vi "参数配置表.vi"() -> ()   [LabVIEW 2016, in "数据传输系统-03.lvlib"]
uses:
  <vilib>/Utility/miscctls.llb/LVPointTypeDef.ctl
  <vilib>/Utility/config.llb/NI_LVConfig.lvlib
  <vilib>/ptbypt/NI_PtbyPt.lvlib
panel:
  in  "数据库类型":enum16{"Access", "SQLite"}(ring)
  in  "应用环境":enum16{"STD", "GB212"}(ring)
  in  "屏蔽维护数据":bool
  in  "数据发送延时时间/s":i32
  in  "判断数据反馈":enum16{"非严格判断", "严格判断", "不判断"}(ring)
  in  "仪器参数发送":bool
  in  "地表水/污染源":bool
  in  "间隔时间/分钟":i32
  in  "数据发送通道":enum16{"TCP", "VISA"}(ring)
  in  "数据发送协议":enum16{"2005-212协议", "2017-212协议"}(ring)=enum."2017-212协议"
  in  "数据触发上传方式":enum16{"出数即刻发送", "间隔时间发送", "整点发送"}(ring)
  in  "数据组合发送":bool
  in  "日志、参数发送":bool
  in  "2011发送":bool
  in  "返回":bool
  out "配置表格":string[][](table)
  in  "参数数值":T1={"CODMn"=TRUE, "CODCr"=TRUE, "DO"=TRUE, "铜"=TRUE, "PH"=TRUE, "氨氮"=TRUE, "比电导率"=TRUE, "水温"=TRUE, "COD"=TRUE, "浊度"=TRUE, "总氮"=TRUE, "总磷"=TRUE, "叶绿素a"=TRUE, "藻密度"=TRUE, "水位"=TRUE, "流速"=TRUE, "瞬时流量"=TRUE, "累积流量"=TRUE, "亚硝氮"=TRUE, "硫化物"=TRUE, "ORP"=TRUE, "铅"=TRUE, "镉"=TRUE, "锌"=TRUE, "镍"=TRUE, "锰"=TRUE, "汞"=TRUE, "气温"=TRUE, "气压"=TRUE, "风速"=TRUE, "风向"=TRUE, "盐度"=TRUE, "磷酸盐"=TRUE, "硝氮"=TRUE}
  # "因子编码，单位配置，上传功能码，小时、质控数据上传触发方式"
  # "参数配置"
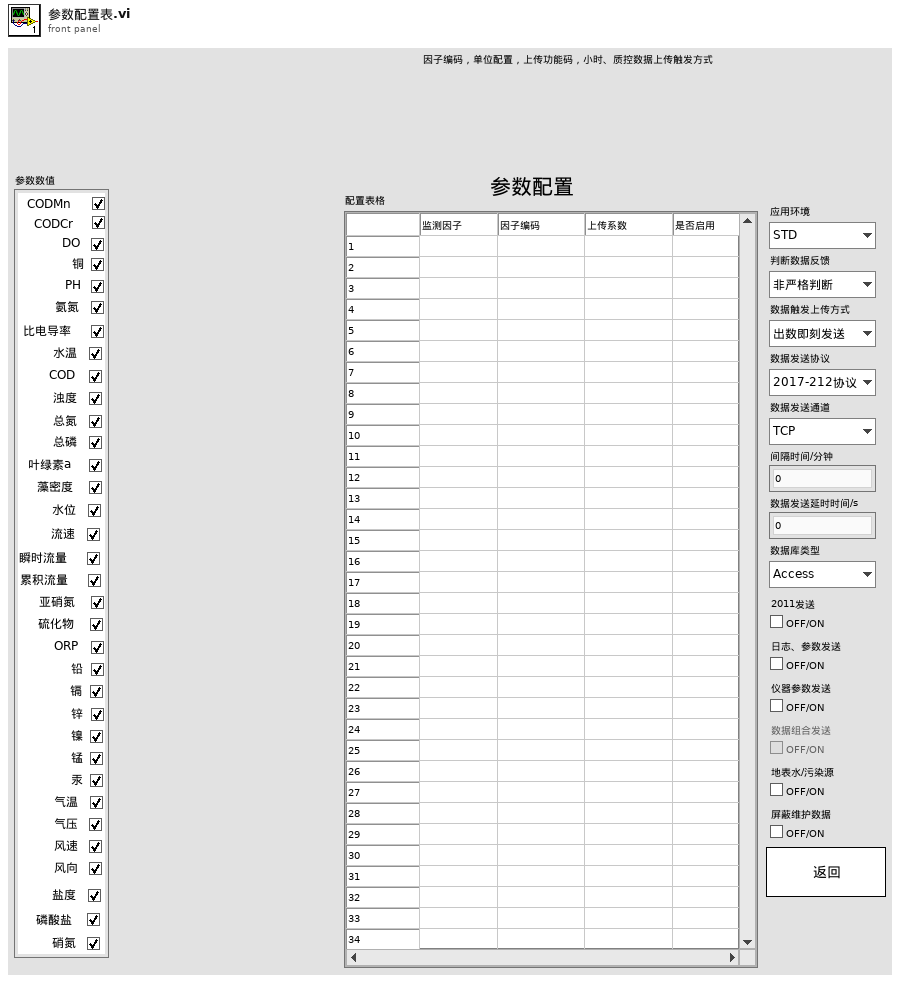
[diagram p1: front panel]
types:
  T1 = cluster{"CODMn":bool, "CODCr":bool, "DO":bool, "铜":bool, "PH":bool, "氨氮":bool, "比电导率":bool, "水温":bool, "COD":bool, "浊度":bool, "总氮":bool, "总磷":bool, "叶绿素a":bool, "藻密度":bool, "水位":bool, "流速":bool, "瞬时流量":bool, "累积流量":bool, "亚硝氮":bool, "硫化物":bool, "ORP":bool, "铅":bool, "镉":bool, "锌":bool, "镍":bool, "锰":bool, "汞":bool, "气温":bool, "气压":bool, "风速":bool, "风向":bool, "盐度":bool, "磷酸盐":bool, "硝氮":bool}
  T2 = typedef "LVPointTypeDef.ctl" = cluster{"Horizontal":i16, "Vertical":i16}
  T3 = typedef "NI_LVConfig.lvlib/Config Data RefNum.ctl" = refnum<k1>
  T4 = cluster{"[0]":string, "[1]":string, "[2]":string, "[3]":string, "[4]":string, "[5]":string, "[6]":string, "[7]":string, "[8]":string, "[9]":string, "[10]":string, "[11]":string, "[12]":string, "[13]":string, "[14]":string, "[15]":string, "[16]":string, "[17]":string, "[18]":string, "[19]":string, "[20]":string, "[21]":string, "[22]":string, "[23]":string, "[24]":string, "[25]":string, "[26]":string, "[27]":string, "[28]":string, "[29]":string, "[30]":string, "[31]":string, "[32]":string, "[33]":string}
  T5 = enum8{"Enabled", "Disabled", "Disabled and Grayed Out"}
  T6 = typedef "LVRowAndColumnTypeDef.ctl" = cluster{"Row":i32, "Column":i32}
  T7 = cluster{"[0]":string, "[1]":string, "[2]":string, "[3]":string, "[4]":string, "[5]":string}
  T8 = cluster{"[0]":string, "[1]":string, "[2]":string, "[3]":string, "[4]":string, "[5]":string, "[6]":string, "[7]":string, "[8]":string, "[9]":string, "[10]":string, "[11]":string}
  T9 = cluster{"[0]":string, "[1]":string, "[2]":string, "[3]":string, "[4]":string, "[5]":string, "[6]":string, "[7]":string, "[8]":string, "[9]":string, "[10]":string, "[11]":string, "[12]":string}
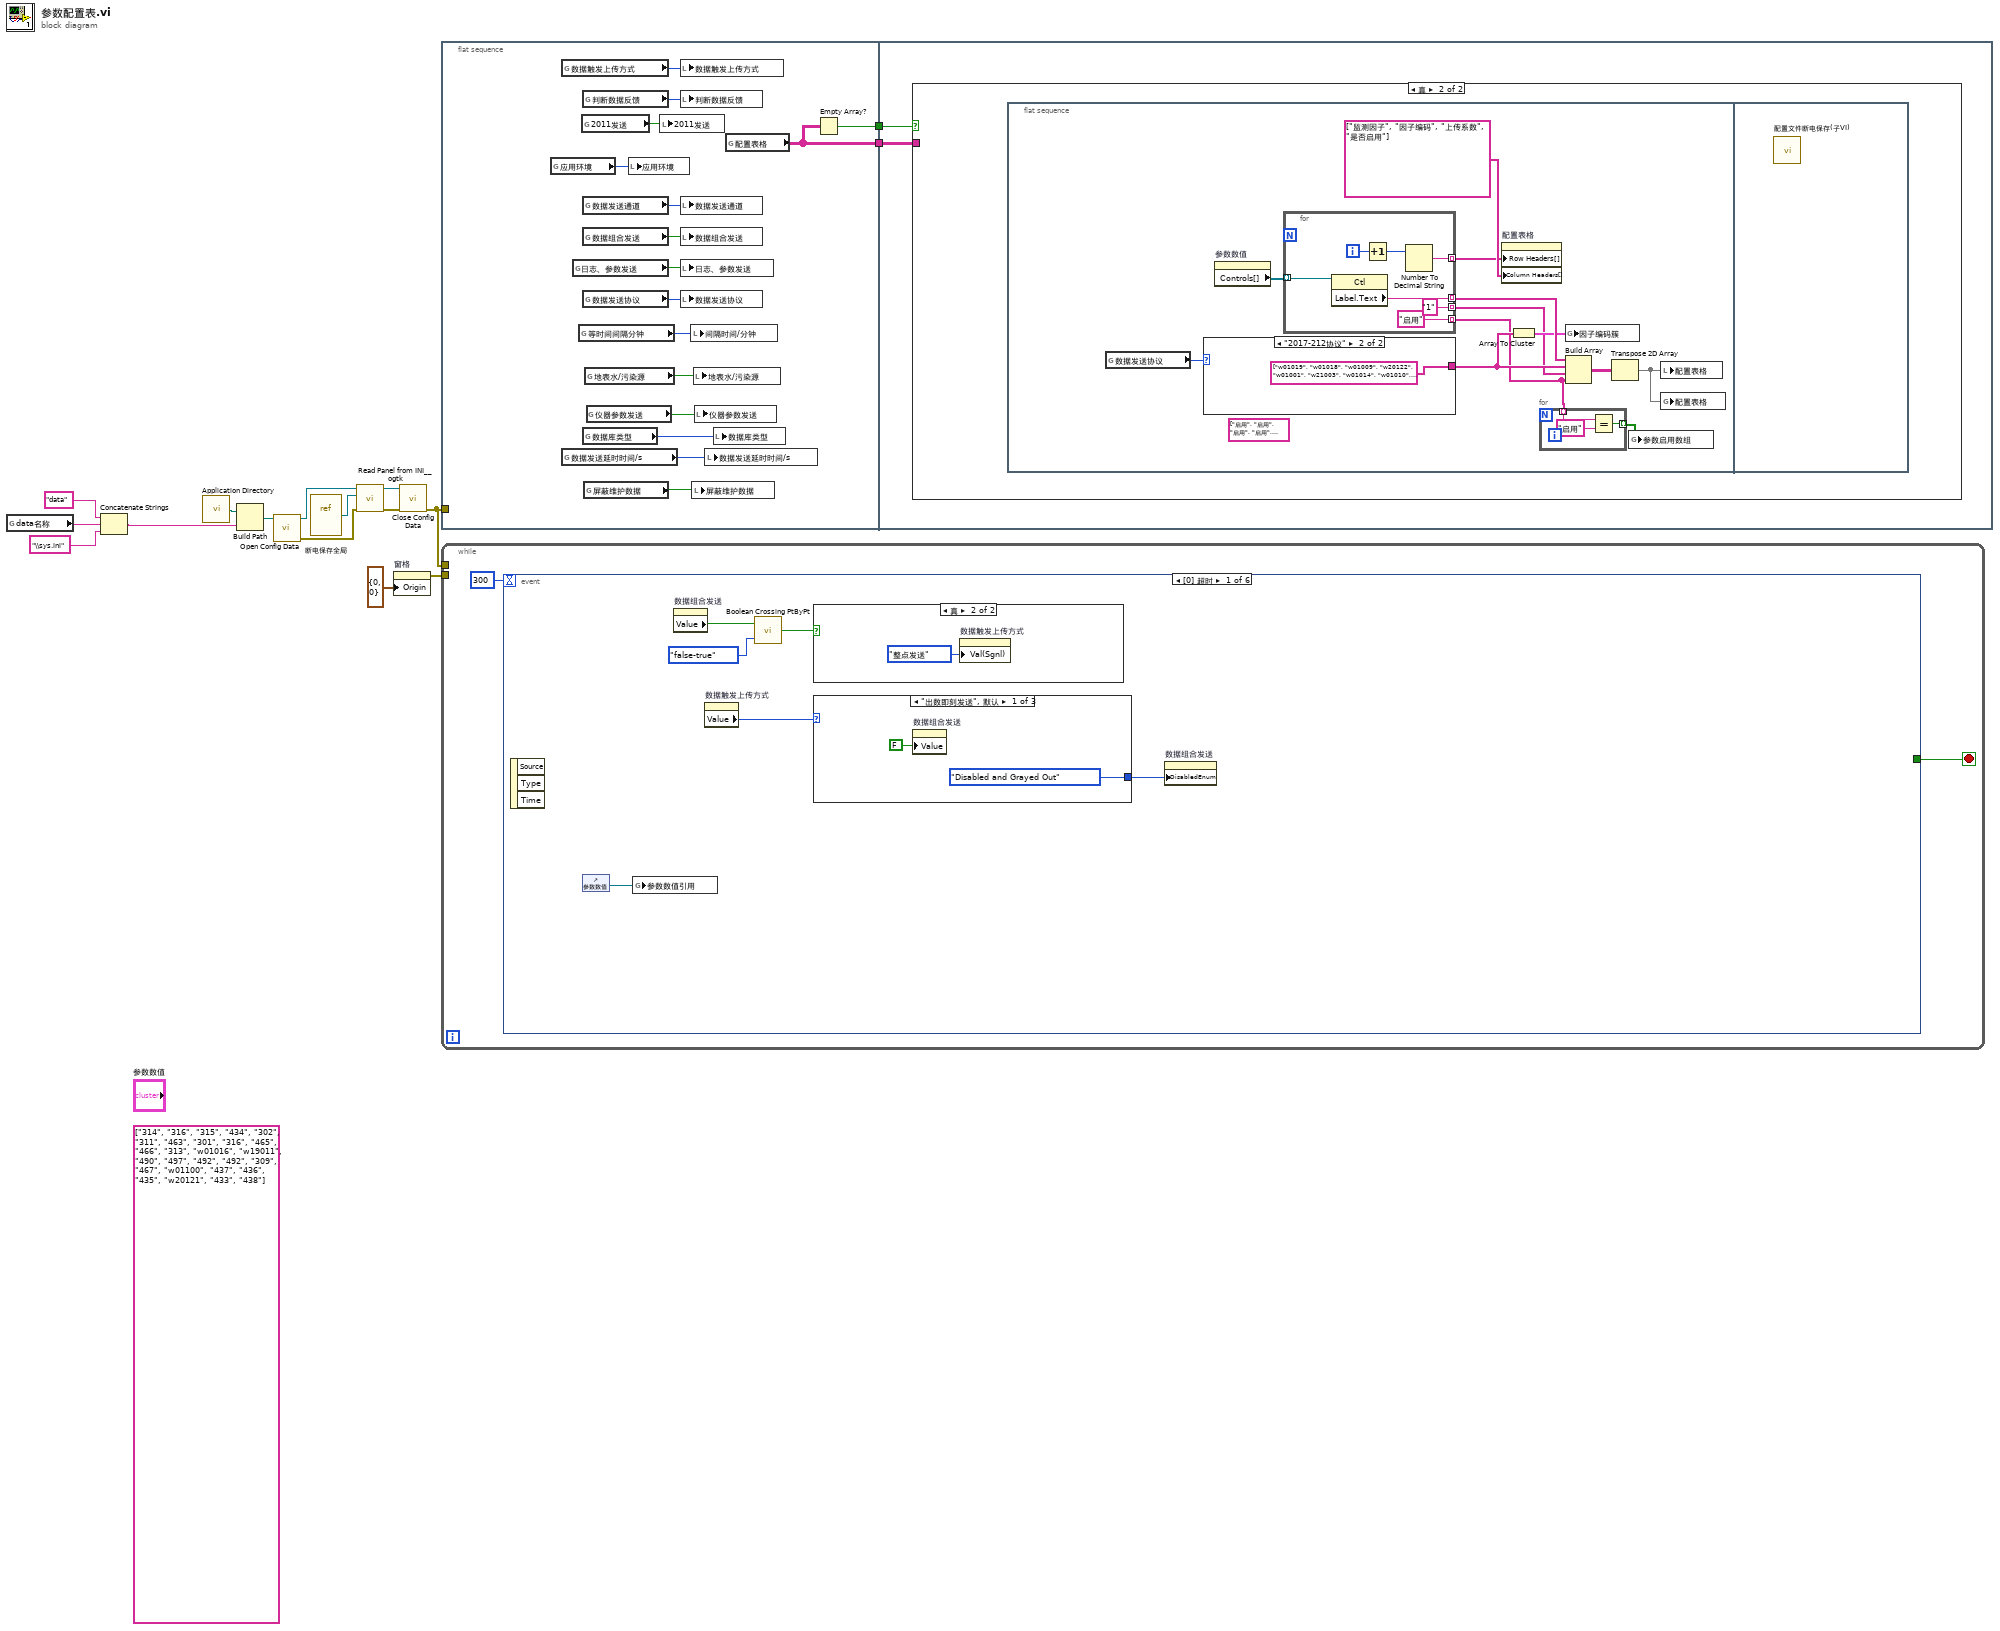
[diagram p0: block diagram]
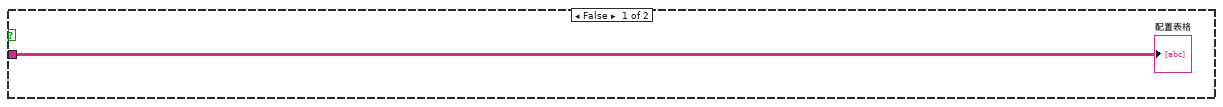
[diagram p2: hidden frame]
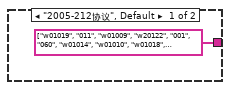
[diagram p3: hidden frame]
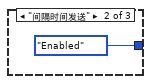
[diagram p5: hidden frame]
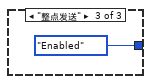
[diagram p6: hidden frame]
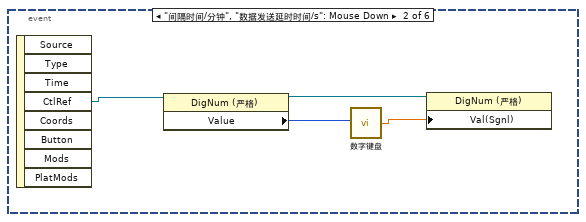
[diagram p7: hidden frame]
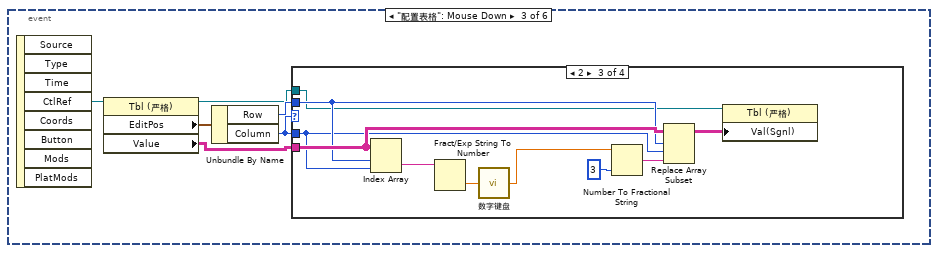
[diagram p8: hidden frame]
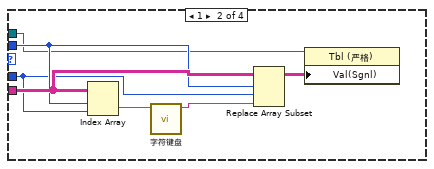
[diagram p10: hidden frame]
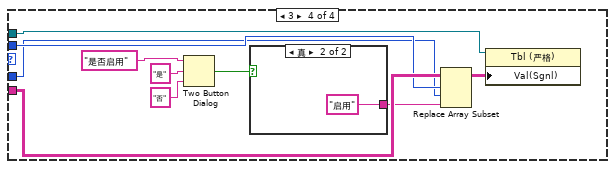
[diagram p11: hidden frame]
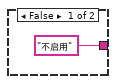
[diagram p12: hidden frame]
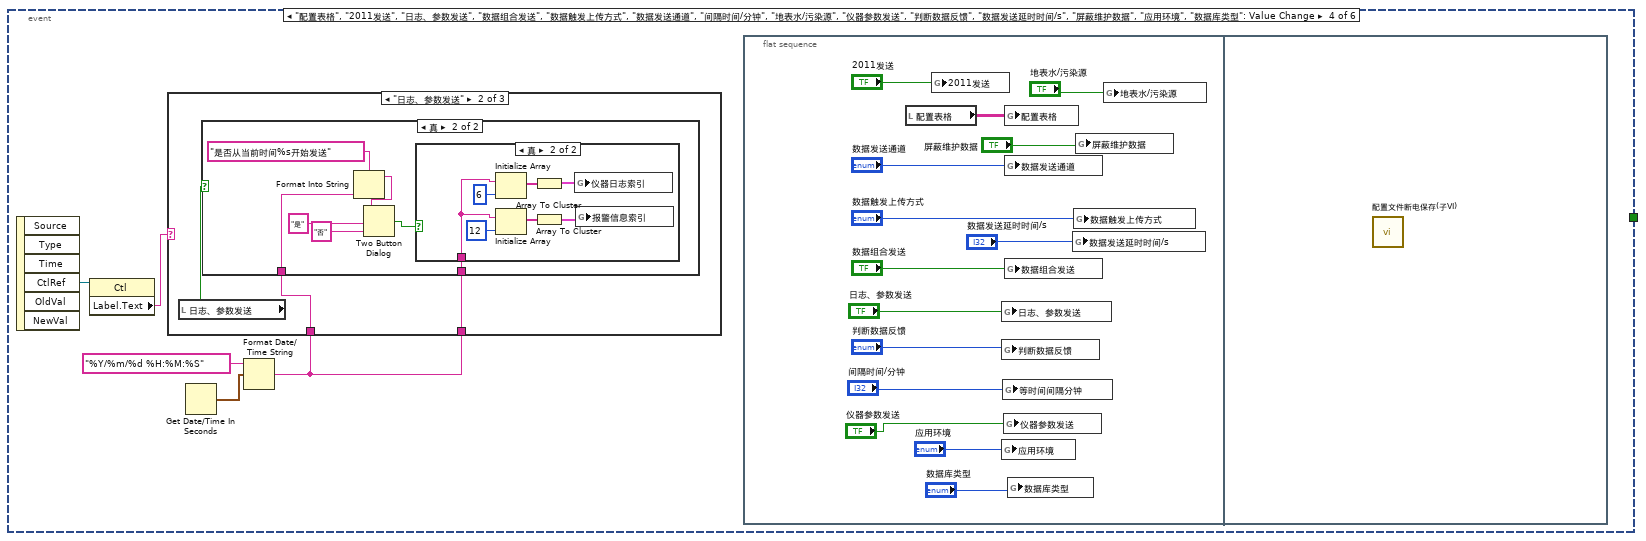
[diagram p13: hidden frame]
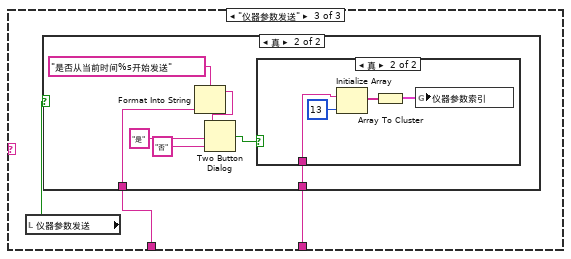
[diagram p17: hidden frame]
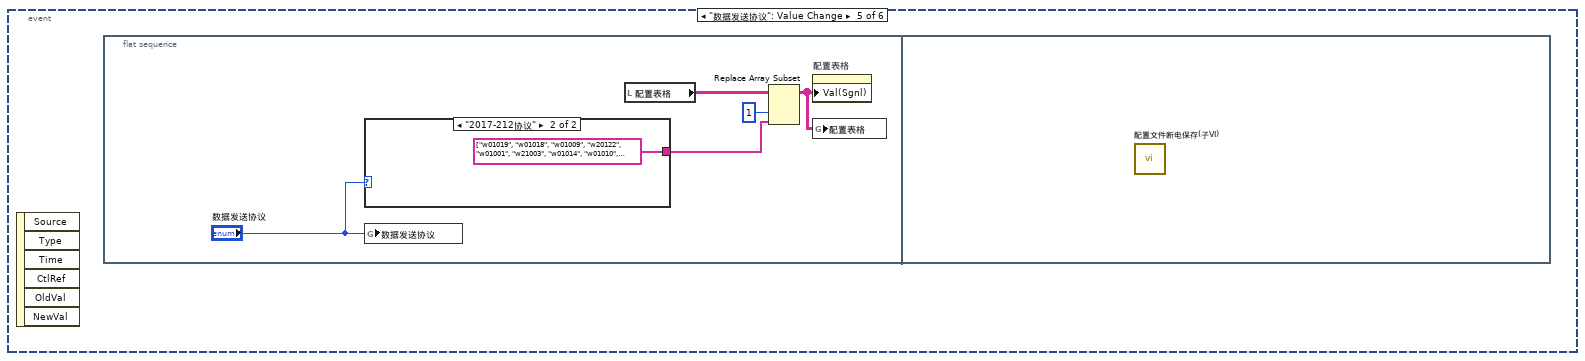
[diagram p20: hidden frame]
diagram:
  (unwired) string[] ["314", "316", "315", "434", "302", "311", "463", "301", "316", "465", "466", "313", "w01016", "w19011", "490", "497", "492", "492", "309", "467", "w01100", "437", "436", "435", "w20121", "433", "438"]
  n1 = global read "断电保存全局.vi" "data名称"() -> (w3:string)
  n2 = Concatenate Strings("data" ("名称或相对路径"), w3, "\\sys.ini" ("名称或相对路径")) -> (w1:string)
  n3 = call <vilib>:"Application Directory.vi"() -> ("Application Directory"=w12:path)
  n4 = Build Path(base path=w12, name or relative path=w1) -> (appended path=w11:path)
  n5 = call <vilib>:"Open Config Data.vi"("configuration file path"=w11) -> ("error out"=w16:errorcluster, "refnum"=w15:T3)  [unwired: 8 in, 1 out]
  n6 = vi-ref "断电保存全局.vi"() -> (w14:refnum<vi>)
  n7 = call <userlib>:"Read Panel from INI__ogtk.vi"("error in (no error)"=w16, "VI ref"=w14, "refnum"=w15) -> ("error out"=w10:errorcluster, "refnum out"=w13:T3)  [unwired: 7 in]
  n8 = property on="窗格" class="Pane"("Origin"=T2 {"Horizontal"=0, "Vertical"=0} ("原点")) -> (error out=w8:errorcluster)  [unwired: 2 in, 1 out]
  n9 = call <vilib>:"Close Config Data.vi"("error in (no error)"=w10, "refnum"=w13) -> ("error out"=w9:errorcluster)  [unwired: 8 in, 1 out]
  n10 = flat-sequence {
    tunnel: w9 -> [_]
    tunnel: [w25] -> w6
    tunnel: [w24] -> w5
    tunnel: w6 -> [w34]
    tunnel: w5 -> [w33]
    frame #0 {
      n11 = global read "断电保存全局.vi" "应用环境"() -> (w18:enum16{"STD", "GB212"})
      n12 = global read "断电保存全局.vi" "数据触发上传方式"() -> (w28:enum16{"出数即刻发送", "间隔时间发送", "整点发送"})
      n13 = global read "断电保存全局.vi" "数据发送延时时间/s"() -> (w20:i32)
      n14 = global read "断电保存全局.vi" "日志、参数发送"() -> (w30:bool)
      n15 = global read "断电保存全局.vi" "等时间间隔分钟"() -> (w23:i32)
      n16 = global read "断电保存全局.vi" "2011发送"() -> (w32:bool)
      n17 = global read "断电保存全局.vi" "判断数据反馈"() -> (w31:enum16{"非严格判断", "严格判断", "不判断"})
      n18 = global read "断电保存全局.vi" "数据发送通道"() -> (w27:enum16{"TCP", "VISA"})
      n19 = global read "断电保存全局.vi" "数据组合发送"() -> (w29:bool)
      n20 = global read "断电保存全局.vi" "数据发送协议"() -> (w26:enum16{"2005-212协议", "2017-212协议"})
      n21 = global read "断电保存全局.vi" "数据库类型"() -> (w17:enum16{"Access", "SQLite"})
      n22 = global read "断电保存全局.vi" "屏蔽维护数据"() -> (w19:bool)
      n23 = global read "断电保存全局.vi" "地表水/污染源"() -> (w22:bool)
      n24 = global read "断电保存全局.vi" "仪器参数发送"() -> (w21:bool)
      n25 = local write "应用环境"(w18) -> ()
      n26 = local write "2011发送"(w32) -> ()
      n27 = local write "数据触发上传方式"(w28) -> ()
      n28 = local write "判断数据反馈"(w31) -> ()
      n29 = local write "数据发送通道"(w27) -> ()
      n30 = local write "数据组合发送"(w29) -> ()
      n31 = local write "日志、参数发送"(w30) -> ()
      n32 = local write "数据发送协议"(w26) -> ()
      n33 = local write "间隔时间/分钟"(w23) -> ()
      n34 = local write "屏蔽维护数据"(w19) -> ()
      n35 = local write "地表水/污染源"(w22) -> ()
      n36 = local write "仪器参数发送"(w21) -> ()
      n37 = local write "数据发送延时时间/s"(w20) -> ()
      n38 = local write "数据库类型"(w17) -> ()
      n39 = global read "断电保存全局.vi" "配置表格"() -> (w24:string[][])
      n40 = Empty Array?(array=w24) -> (empty?=w25:bool)
    }
    frame #1 {
      n41 = case shown="真" w34 {
        tunnel: w33 -> [w35 _]
        frame False {
          "配置表格" <- w35
        }
        frame True {
          n42 = flat-sequence {
            frame #0 {
              (unwired) string[] ["启用", "启用", "启用", "启用", "启用", "启用", "启用", "启用", "启用", "启用", "启用", "启用", "启用", "启用", "启用", "启用", "启用", "启用", "启用", "启用", "启用", "启用", "启用", "启用", "启用", "启用", "启用"]
              n43 = global read "断电保存全局.vi" "数据发送协议"() -> (w41:enum16{"2005-212协议", "2017-212协议"})
              n44 = case shown="\"2017-212协议\"" w41 {
                tunnel: [string[] ["w01019", "011", "w01009", "w20122", "001", "060", "w01014", "w01010", "w01018", "w01003", "065", "101", "w01016", "w19011", "e01201", "e01202", "B01", "e01204", "w21006", "w21019", "w01100", "w20120", "w20115", "w20123", "w20121", "w20124", "w20111"] string[] ["w01019", "w01018", "w01009", "w20122", "w01001", "w21003", "w01014", "w01010", "w01018", "w01003", "w21001", "w21011", "w01016", "w19011", "e01201", "e01202", "e01203", "e01204", "w21006", "w21019", "w01100", "w20120", "w20115", "w20123", "w20121", "w20124", "w20111", "a01001", "a01006", "a01007", "a01008", "w01002", "w21015", "w21007"]] -> w39
                frame "2005-212协议", Default {
                }
                frame "2017-212协议" {
                }
              }
              n45 = property on="参数数值" class="Clust (严格)"() -> ("Controls[]"=w43:refnum<vi>[])  [unwired: 2 in, 2 out]
              n46 = for {
                tunnel: w43 -> [w59] mode=indexing
                tunnel: [w58] -> w45 mode=indexing
                tunnel: [w56] -> w44 mode=indexing
                tunnel: ["1"] -> w38 mode=indexing
                tunnel: ["启用"] -> w36 mode=indexing
                i -> [w57]
                n47 = property class="Ctl"(reference=w59) -> ("Label.Text"=w58:string)  [unwired: 1 in, 2 out]
                n48 = Increment(x=w57) -> (x+1=w55:i32)
                n49 = Number To Decimal String(number=w55) -> (decimal integer string=w56:string)  [unwired: 1 in]
              }
              n50 = property on="配置表格" class="Tbl (严格)"("Row Headers[]"=w44, "Column Headers[]"=string[] ["监测因子", "因子编码", "上传系数", "是否启用"]) -> ()  [unwired: 2 in, 2 out]
              n51 = Array To Cluster(array=w39) -> (cluster=w40:T4)
              n52 = for {
                tunnel: w36 -> [w50] mode=indexing
                tunnel: [w48] -> w37 mode=indexing
                n53 = Equal?(x=w50, y="启用") -> (x = y?=w48:bool)
              }
              n54 = global write "断电保存全局.vi" "因子编码簇"(w40) -> ()
              n55 = Build Array(w45, w39, w38, w36) -> (w47:string[][])
              n56 = Transpose 2D Array(2D array=w47) -> (transposed array=w42:string[][])
              n57 = global write "断电保存全局.vi" "参数启用数组"(w37) -> ()
              n58 = local write "配置表格"(w42) -> ()
              n59 = global write "断电保存全局.vi" "配置表格"(w42) -> ()
            }
            frame #1 {
              n60 = call "配置文件断电保存(子VI).vi"() -> ()  [unwired: 12 in]
            }
          }
        }
      }
    }
  }
  n61 = while {
    tunnel: w9 -> [_]
    tunnel: w8 -> [_]
    stop <- w60 stop-if-true
    n62 = event shown="[0] 超时" {
      selector: _ -> [_ _ _ _ _ _]
      dyn-events: _ -> [_ _ _ _ _ _]
      timeout: 300 -> [_ _ _ _ _ _]
      tunnel: [_ _ _ _ _ TRUE] -> w60
      event Timeout {
        n63 = event-data() -> ()  [unwired: 1 in, 3 out]
        n64 = control-ref of="参数数值"() -> (w62:refnum<vi>)
        n65 = global write "断电保存全局.vi" "参数数值引用"(w62) -> ()
        n66 = property on="数据组合发送" class="Bool (严格)"() -> ("Value"=w65:bool)  [unwired: 2 in, 2 out]
        n67 = property on="数据触发上传方式" class="Enum (严格)"() -> ("Value"=w67:enum16{"出数即刻发送", "间隔时间发送", "整点发送"})  [unwired: 2 in, 2 out]
        n68 = call <vilib>:"Boolean Crossing PtByPt.vi"("direction"=enum16{"either", "false-true", "true-false"}."false-true", "input"=w65) -> ("crossing"=w63:bool)  [unwired: 1 in]
        n69 = case shown="真" w63 {
          frame False {
          }
          frame True {
            n70 = property on="数据触发上传方式" class="Enum (严格)"("Val(Sgnl)"=enum16{"出数即刻发送", "间隔时间发送", "整点发送"}."整点发送" ("值(信号)")) -> ()  [unwired: 2 in, 2 out]
          }
        }
        n71 = case shown="\"出数即刻发送\", 默认" w67 {
          tunnel: [T5."Disabled and Grayed Out" ("禁用") T5."Enabled" ("禁用") T5."Enabled" ("禁用")] -> w66
          frame "出数即刻发送", Default {
            n72 = property on="数据组合发送" class="Bool (严格)"("Value"=FALSE ("值(信号)")) -> ()  [unwired: 2 in, 2 out]
          }
          frame "间隔时间发送" {
          }
          frame "整点发送" {
          }
        }
        n73 = property on="数据组合发送" class="Bool (严格)"("DisabledEnum"=w66) -> ()  [unwired: 2 in, 2 out]
      }
      event "间隔时间/分钟", "数据发送延时时间/s": Mouse Down {
        n74 = event-data() -> ("CtlRef"=w76:refnum<vi>)  [unwired: 1 in, 7 out]
        n75 = property class="DigNum (严格)"(reference=w76) -> (reference out=w74:refnum<vi>, "Value"=w75:i32)  [unwired: 1 in, 1 out]
        n76 = call "数字键盘.vi"("OldNumber"=w75) -> ("NewNumber"=w73:sgl)
        n77 = property class="DigNum (严格)"(reference=w74, "Val(Sgnl)"=w73) -> ()  [unwired: 1 in, 2 out]
      }
      event "配置表格": Mouse Down {
        n78 = event-data() -> ("CtlRef"=w82:refnum<vi>)  [unwired: 1 in, 7 out]
        n79 = property class="Tbl (严格)"(reference=w82) -> (reference out=w78:refnum<vi>, "EditPos"=w81:T6, "Value"=w80:string[][])  [unwired: 1 in, 1 out]
        n80 = Unbundle By Name(w81) -> ("Row"=w79:i32, "Column"=w77:i32)
        n81 = case shown="2" w77 {
          tunnel: w80 -> [_ w88 w99 w103]
          tunnel: w79 -> [_ w87 w98 w102]
          tunnel: w77 -> [_ w86 w97 w101]
          tunnel: w78 -> [_ w84 w96 w104]
          frame 0, Default {
          }
          frame 1 {
            n82 = Index Array(array=w88, index (row)=w87, index (col)=w86) -> (element=w89:string)
            n83 = call "字符键盘.vi"("原值"=w89) -> ("x+y"=w85:string)  [unwired: 10 in]
            n84 = Replace Array Subset(array=w88, new element=w85, index (row)=w87, index (col)=w86) -> (w83:string[][])
            n85 = property class="Tbl (严格)"(reference=w84, "Val(Sgnl)"=w83) -> ()  [unwired: 1 in, 2 out]
          }
          frame 2 {
            n86 = Index Array(array=w99, index (row)=w98, index (col)=w97) -> (element=w94:string)
            n87 = Fract/Exp String To Number(string=w94) -> (number=w93:dbl)  [unwired: 3 in, 1 out]
            n88 = call "数字键盘.vi"("OldNumber"=w93) -> ("NewNumber"=w92:sgl)
            n89 = Number To Fractional String(number=w92, precision (6)=i16 3 ("精度(6)")) -> (F-format string=w91:string)  [unwired: 2 in]
            n90 = Replace Array Subset(array=w99, new element=w91, index (row)=w98, index (col)=w97) -> (w95:string[][])
            n91 = property class="Tbl (严格)"(reference=w96, "Val(Sgnl)"=w95) -> ()  [unwired: 1 in, 2 out]
          }
          frame 3 {
            n92 = Two Button Dialog(message="是否启用" ("消息"), 1:"否" ("F按钮名称（“取消”）"), 2:"是" ("T按钮名称（“确定”）")) -> (T button?=w106:bool)
            n93 = case shown="真" w106 {
              tunnel: ["不启用" "启用"] -> w100
              frame False {
              }
              frame True {
              }
            }
            n94 = Replace Array Subset(array=w103, new element=w100, index (row)=w102, index (col)=w101) -> (w105:string[][])
            n95 = property class="Tbl (严格)"(reference=w104, "Val(Sgnl)"=w105) -> ()  [unwired: 1 in, 2 out]
          }
        }
      }
      event "配置表格", "2011发送", "日志、参数发送", "数据组合发送", "数据触发上传方式", "数据发送通道", "间隔时间/分钟", "地表水/污染源", "仪器参数发送", "判断数据反馈", "数据发送延时时间/s", "屏蔽维护数据", "应用环境", "数据库类型": Value Change {
        n96 = event-data() -> ("CtlRef"=w116:refnum<vi>)  [unwired: 1 in, 5 out]
        n97 = property class="Ctl"(reference=w116) -> ("Label.Text"=w115:string)  [unwired: 1 in, 2 out]
        n98 = Get Date/Time In Seconds() -> (seconds since 1Jan1904=w114:timestamp)
        n99 = Format Date/Time String(time format string (%c)="%Y/%m/%d %H:%M:%S" ("时间格式字符串(%c)"), seconds (now)=w114) -> (date/time string=w112:string)  [unwired: 1 in]
        n100 = case shown="\"日志、参数发送\"" w115 {
          tunnel: w112 -> [_ w118 w135]
          tunnel: w112 -> [_ w117 w134]
          frame "假", Default {
          }
          frame "日志、参数发送" {
            n101 = local read "日志、参数发送"() -> (w119:bool)
            n102 = case shown="真" w119 {
              tunnel: w118 -> [_ w123]
              tunnel: w117 -> [_ w121]
              frame False {
              }
              frame True {
                n103 = Format Into String(format string="是否从当前时间%s开始发送" ("消息"), w121) -> (resulting string=w120:string)  [unwired: 2 in, 1 out]
                n104 = Two Button Dialog(message=w120, 1:"否" ("F按钮名称（“取消”）"), 2:"是" ("T按钮名称（“确定”）")) -> (T button?=w124:bool)
                n105 = case shown="真" w124 {
                  tunnel: w123 -> [_ w127]
                  frame False {
                  }
                  frame True {
                    n106 = Initialize Array(w127, 6 ("维数大小")) -> (w133:string[])
                    n107 = Initialize Array(w127, 12 ("维数大小")) -> (w129:string[])
                    n108 = Array To Cluster(array=w133) -> (cluster=w131:T7)
                    n109 = Array To Cluster(array=w129) -> (cluster=w128:T8)
                    n110 = global write "全局 时间2.vi" "仪器日志索引"(w131) -> ()
                    n111 = global write "全局 时间2.vi" "报警信息索引"(w128) -> ()
                  }
                }
              }
            }
          }
          frame "仪器参数发送" {
            n112 = local read "仪器参数发送"() -> (w136:bool)
            n113 = case shown="真" w136 {
              tunnel: w135 -> [_ w140]
              tunnel: w134 -> [_ w138]
              frame False {
              }
              frame True {
                n114 = Format Into String(format string="是否从当前时间%s开始发送" ("消息"), w138) -> (resulting string=w137:string)  [unwired: 2 in, 1 out]
                n115 = Two Button Dialog(message=w137, 1:"否" ("F按钮名称（“取消”）"), 2:"是" ("T按钮名称（“确定”）")) -> (T button?=w141:bool)
                n116 = case shown="真" w141 {
                  tunnel: w140 -> [_ w144]
                  frame False {
                  }
                  frame True {
                    n117 = Initialize Array(w144, 13 ("维数大小")) -> (w147:string[])
                    n118 = Array To Cluster(array=w147) -> (cluster=w145:T9)
                    n119 = global write "全局 时间2.vi" "仪器参数索引"(w145) -> ()
                  }
                }
              }
            }
          }
        }
        n120 = flat-sequence {
          frame #0 {
            n121 = local read "配置表格"() -> (w161:string[][])
            n122 = global write "断电保存全局.vi" "2011发送"("2011发送") -> ()
            n123 = global write "断电保存全局.vi" "日志、参数发送"("日志、参数发送") -> ()
            n124 = global write "断电保存全局.vi" "判断数据反馈"("判断数据反馈") -> ()
            n125 = global write "断电保存全局.vi" "应用环境"("应用环境") -> ()
            n126 = global write "断电保存全局.vi" "等时间间隔分钟"("间隔时间/分钟") -> ()
            n127 = global write "断电保存全局.vi" "仪器参数发送"("仪器参数发送") -> ()
            n128 = global write "断电保存全局.vi" "配置表格"(w161) -> ()
            n129 = global write "断电保存全局.vi" "数据发送通道"("数据发送通道") -> ()
            n130 = global write "断电保存全局.vi" "数据组合发送"("数据组合发送") -> ()
            n131 = global write "断电保存全局.vi" "数据库类型"("数据库类型") -> ()
            n132 = global write "断电保存全局.vi" "数据发送延时时间/s"("数据发送延时时间/s") -> ()
            n133 = global write "断电保存全局.vi" "数据触发上传方式"("数据触发上传方式") -> ()
            n134 = global write "断电保存全局.vi" "屏蔽维护数据"("屏蔽维护数据") -> ()
            n135 = global write "断电保存全局.vi" "地表水/污染源"("地表水/污染源") -> ()
          }
          frame #1 {
            n136 = call "配置文件断电保存(子VI).vi"() -> ()  [unwired: 12 in]
          }
        }
      }
      event "数据发送协议": Value Change {
        n137 = event-data() -> ()  [unwired: 1 in, 6 out]
        n138 = flat-sequence {
          frame #0 {
            n139 = case shown="\"2017-212协议\"" "数据发送协议" {
              tunnel: [string[] ["w01019", "011", "w01009", "w20122", "001", "060", "w01014", "w01010", "w01018", "w01003", "065", "101", "w01016", "w19011", "e01201", "e01202", "B01", "e01204", "w21006", "w21019", "w01100", "w20120", "w20115", "w20123", "w20121", "w20124", "w20111"] string[] ["w01019", "w01018", "w01009", "w20122", "w01001", "w21003", "w01014", "w01010", "w01018", "w01003", "w21001", "w21011", "w01016", "w19011", "e01201", "e01202", "e01203", "e01204", "w21006", "w21019", "w01100", "w20120", "w20115", "w20123", "w20121", "w20124", "w20111"]] -> w164
              frame "2005-212协议", Default {
              }
              frame "2017-212协议" {
              }
            }
            n140 = global write "断电保存全局.vi" "数据发送协议"("数据发送协议") -> ()
            n141 = local read "配置表格"() -> (w165:string[][])
            n142 = Replace Array Subset(array=w165, new element=w164, index (col)=1 ("禁用的索引 (列)")) -> (w162:string[][])  [unwired: 1 in]
            n143 = property on="配置表格" class="Tbl (严格)"("Val(Sgnl)"=w162) -> ()  [unwired: 2 in, 2 out]
            n144 = global write "断电保存全局.vi" "配置表格"(w162) -> ()
          }
          frame #1 {
            n145 = call "配置文件断电保存(子VI).vi"() -> ()  [unwired: 12 in]
          }
        }
      }
      event "返回": Value Change; Panel Close {
        n146 = event-data() -> ()  [unwired: 1 in, 3 out]
      }
    }
  }
